vi "UTILITY 1D DBL to 1D String.vi"(7 "DBL?":bool=TRUE, 11 "1D DBL":dbl[](array[numeric])) -> (3 "1D String":string[](array[string]))   [LabVIEW 2016]
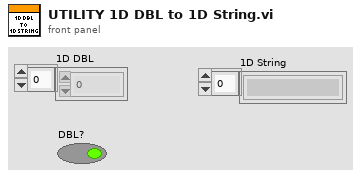
[diagram p1: front panel]
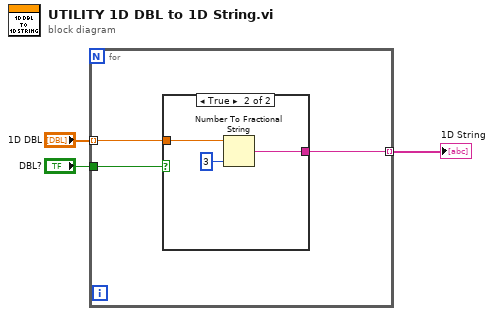
[diagram p0: block diagram]
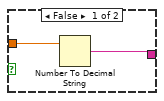
[diagram p2: hidden frame]
diagram:
  n1 = for {
    tunnel: "1D DBL" -> [w6] mode=indexing
    tunnel: [w5] -> w2 mode=indexing
    tunnel: "DBL?" -> [w4]
    n2 = case shown="True" w4 {
      tunnel: w6 -> [w8 w11]
      tunnel: [w7 w10] -> w5
      frame False {
        n3 = Number To Decimal String(number=w8) -> (decimal integer string=w7:string)  [unwired: 1 in]
      }
      frame True {
        n4 = Number To Fractional String(number=w11, precision (6)=i16 3) -> (F-format string=w10:string)  [unwired: 2 in]
      }
    }
  }
  "1D String" <- w2
